vi "rqcBob Configure Ramdom Number Generator.vi"(8 "error in":errorcluster, 10 "rqcBob rndGen.parameters":T2={"value type"=enum."constant", "constant"=0, "num of levels"=0, "levels values"=[0, 0, 0, 0]}, 11 "FPGA reference in":refnum<k20>) -> (0 "error out":errorcluster, 3 "FPGA reference out":refnum<k20>)   [LabVIEW 2019]
uses:
  Shared/Shared FPGA Lib/Shared Logic/Custom Controls/rqc Random Generator.value type.ctl
  <vilib>/Utility/error.llb/Error Cluster From Error Code.vi
  <vilib>/rvi/errors/niLvFpgaAdjustHostInterfaceError.vi
  <vilib>/rvi/interface/nirviReadWriteControl/nirviReadWriteControl.xnode
  NiFpgaLv.dll
  <vilib>/rvi/interface/Simulation/niFpgaSimulationCallBeginRW.vi
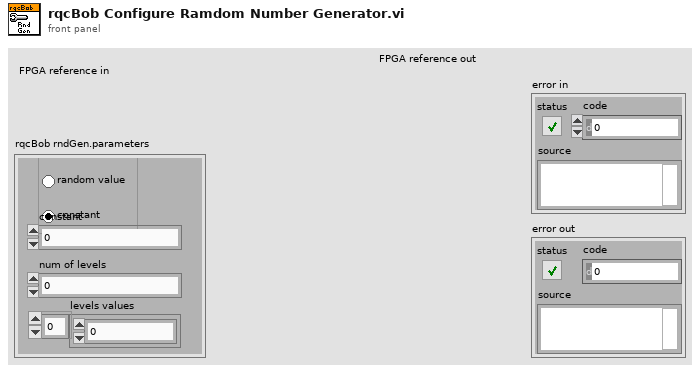
[diagram p1: front panel]
types:
  T1 = typedef "rqc Random Generator.value type.ctl" = enum32{"random value", "constant"}
  T2 = cluster{"value type":T1, "constant":u16, "num of levels":u16, "levels values":u16[]}
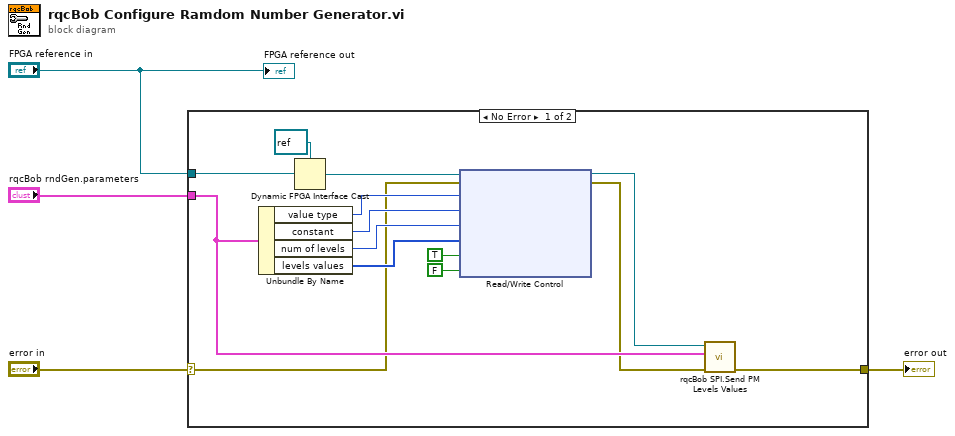
[diagram p0: block diagram]
diagram:
  n1 = case shown="No Error" "error in" {
    selector: "error in" -> [w7 w19]
    tunnel: [w5 w19] -> w2
    tunnel: "FPGA reference in" -> [w17 _]
    tunnel: "rqcBob rndGen.parameters" -> [w9 _]
    frame No Error {
      n2 = Unbundle By Name(w9) -> ("value type"=w13:T1, "constant"=w12:u16, "num of levels"=w11:u16, "levels values"=w10:u16[])
      n3 = Dynamic FPGA Interface Cast(Session In=refnum<k20> refnum ("FPGA Interface"), Type=w17) -> (Session Out=w16:refnum<k20>)
      n4 = xnode "Read/Write Control"("FPGA VI Reference In"=w16, "error in"=w7, "rndGen.value type"=w13, "rndGen.constant"=w12, "rndGen.num of levels"=w11, "rndGen.levels values"=w10, "rndGen.reset"=TRUE, "rndGen.reset"=FALSE) -> ("FPGA VI Reference Out"=w8:refnum<k20>, "error out"=w6:errorcluster)
      n5 = call "rqcBob SPI.Send PM Levels Values.vi"("error in"=w6, "RndGen.parameters"=w9, "Bob FPGA Reference In"=w8) -> ("error out"=w5:errorcluster)  [unwired: 6 in, 2 out]
    }
    frame Error {
    }
  }
  "error out" <- w2
  "FPGA reference out" <- "FPGA reference in"
